vi "Subset_Array_2D.vi"(9 "Subset Array 2D":i8[][](array[numeric])=[[-5, -1, 3], [-4, 0, 4], [-3, 1, 5], [-2, 2, 6]], 10 "Lengths R&C":T1, 11 "Indexs SA":T2={"Rows"=-1, "Columns"=-1} {"Columns" min=-1; "Rows" min=-1}) -> (2 "SubArray 2D":i8[][](array[numeric]))   [LabVIEW 2018]
uses:
  Controls/Rows_Columns.ctl
  Controls/Lengths_Rows_Columns.ctl
panel:
  out "Length Columns":i32
  out "Length Rows":i32
  out "Columns":i32
  out "Rows":i32
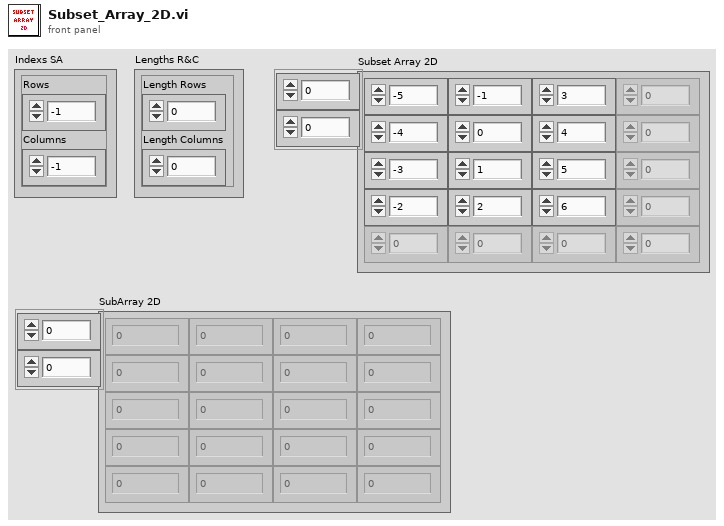
[diagram p1: front panel]
types:
  T1 = typedef "Lengths_Rows_Columns.ctl" = cluster{"Length Rows":i32, "Length Columns":i32}
  T2 = typedef "Rows_Columns.ctl" = cluster{"Rows":i32, "Columns":i32}
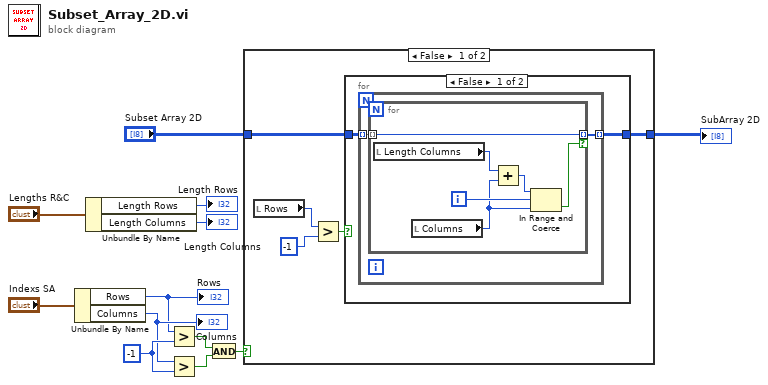
[diagram p0: block diagram]
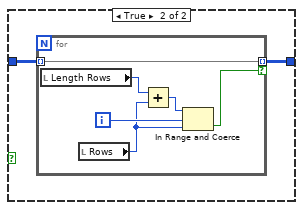
[diagram p2: hidden frame]
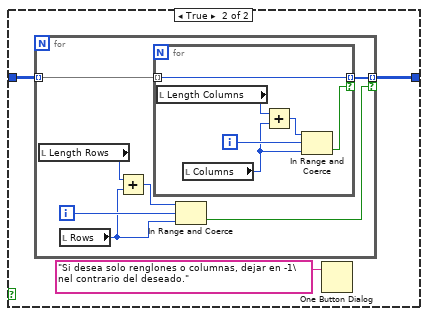
[diagram p3: hidden frame]
diagram:
  w9 = -1 ("y")
  n1 = Unbundle By Name("Indexs SA") -> ("Rows"=w2:i32, "Columns"=w6:i32)
  "Rows" <- w2
  "Columns" <- w6
  n2 = Unbundle By Name("Lengths R&C") -> ("Length Rows"=→"Length Rows":i32, "Length Columns"=→"Length Columns":i32)
  n3 = Greater?(x=w2, y=w9) -> (0:w12:bool)
  n4 = Greater?(x=w6, y=w9) -> (0:w11:bool)
  n5 = And(x=w12, y=w11) -> (x .and. y?=w8:bool)
  n6 = case shown="False" w8 {
    tunnel: "Subset Array 2D" -> [w14 w38]
    tunnel: [w13 w37] -> w7
    frame False {
      n7 = local read "Rows"() -> (w17:i32)
      n8 = Greater?(x=w17, y=-1) -> (0:w15:bool)
      n9 = case shown="False" w15 {
        tunnel: w14 -> [w19 w29]
        tunnel: [w18 w28] -> w13
        frame False {
          n10 = for {
            tunnel: w19 -> [w21] mode=indexing
            tunnel: [w20] -> w18 mode=indexing
            n11 = for {
              tunnel: [w27] -> w20 mode=indexing if=w22
              tunnel: w21 -> [w27] mode=indexing
              i -> [w26]
              n12 = local read "Length Columns"() -> (w25:i32)
              n13 = local read "Columns"() -> (w24:i32)
              n14 = Add(x=w25, y=w24) -> (x+y=w23:i32)
              n15 = In Range and Coerce(upper limit=w23, x=w26, lower limit=w24) -> (In Range?=w22:bool)  [unwired: 1 out]
            }
          }
        }
        frame True {
          n16 = for {
            tunnel: w29 -> [w31] mode=indexing
            tunnel: [w31] -> w28 mode=indexing if=w30
            i -> [w35]
            n17 = local read "Length Rows"() -> (w34:i32)
            n18 = local read "Rows"() -> (w33:i32)
            n19 = Add(x=w34, y=w33) -> (x+y=w32:i32)
            n20 = In Range and Coerce(upper limit=w32, x=w35, lower limit=w33) -> (In Range?=w30:bool)  [unwired: 1 out]
          }
        }
      }
    }
    frame True {
      n21 = for {
        tunnel: w38 -> [w45] mode=indexing
        tunnel: [w44] -> w37 mode=indexing if=w43
        i -> [w42]
        n22 = local read "Length Rows"() -> (w40:i32)
        n23 = local read "Rows"() -> (w39:i32)
        n24 = Add(x=w40, y=w39) -> (x+y=w41:i32)
        n25 = for {
          tunnel: [w51] -> w44 mode=indexing if=w46
          tunnel: w45 -> [w51] mode=indexing
          i -> [w50]
          n26 = local read "Length Columns"() -> (w49:i32)
          n27 = local read "Columns"() -> (w48:i32)
          n28 = Add(x=w49, y=w48) -> (x+y=w47:i32)
          n29 = In Range and Coerce(upper limit=w47, x=w50, lower limit=w48) -> (In Range?=w46:bool)  [unwired: 1 out]
        }
        n30 = In Range and Coerce(upper limit=w41, x=w42, lower limit=w39) -> (In Range?=w43:bool)  [unwired: 1 out]
      }
      n31 = One Button Dialog(message="Si desea solo renglones o columnas, dejar en -1\nel contrario del deseado.") -> ()  [unwired: 1 in, 1 out]
    }
  }
  "SubArray 2D" <- w7
